vi "LV to ITX 2.2 1D.vi"(0 "Commands":string, 5 "filename":path, 7 "Notes":string, 8 "Array name":string, 9 "1D Array":dbl[](array[numeric])) -> ()   [LabVIEW 2016, in "LV to ITX.lvclass"]
uses:
  LV to ITX.lvclass
panel:
  out "String":string
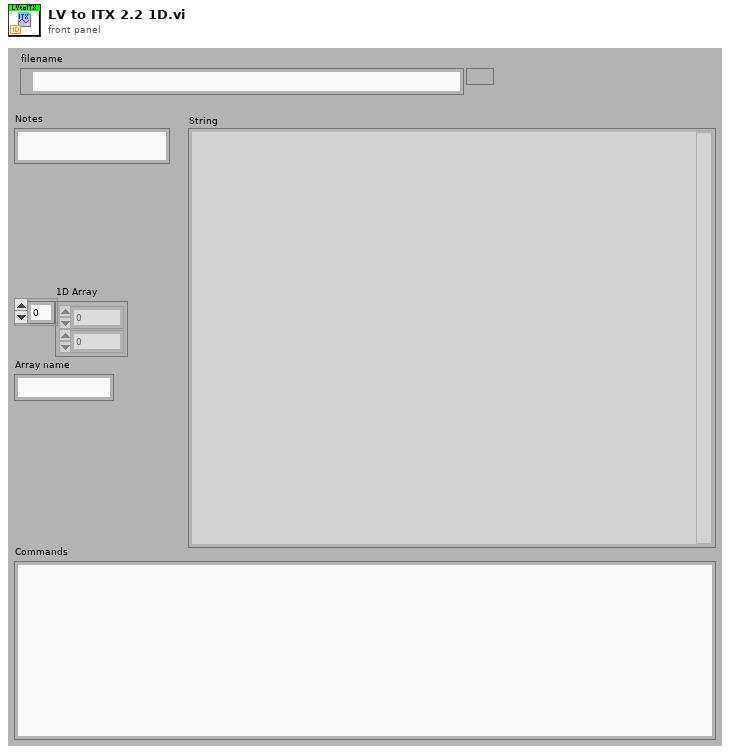
[diagram p1: front panel]
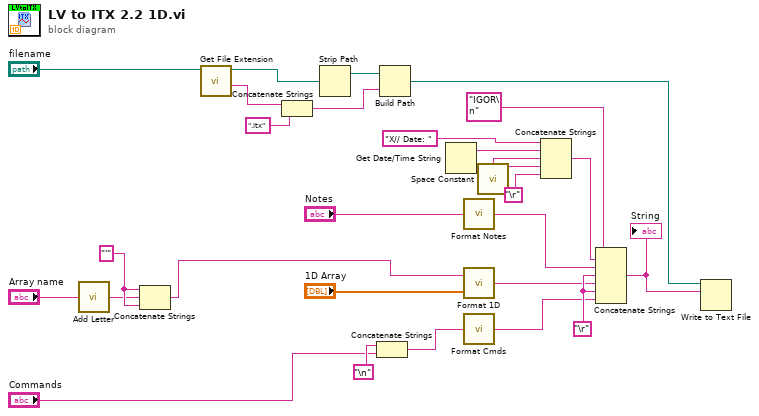
[diagram p0: block diagram]
diagram:
  w3 = "'" ("string")
  w23 = "\r"
  n1 = call "Add Letter.vi"("String"="Array name") -> ("output string"=w2:string)
  n2 = Concatenate Strings(w3, w2, w3) -> (w1:string)
  n3 = call <vilib>:"Get File Extension.vi"("file"="filename") -> ("filename without extension"=w19:string, "dup file"=w15:path)  [unwired: 6 in, 3 out]
  n4 = Concatenate Strings(w19, ".itx") -> (w13:string)
  n5 = Strip Path(path=w15) -> (stripped path=w14:path)  [unwired: 1 out]
  n6 = Concatenate Strings("\n", "Commands") -> (w8:string)
  n7 = Build Path(base path=w14, name or relative path=w13) -> (appended path=w16:path)
  n8 = Get Date/Time String() -> (date string=w27:string, time string=w28:string)  [unwired: 3 in]
  n9 = call "Format Notes.vi"("Notes"="Notes") -> ("String"=w9:string)
  n10 = call "Format 1D.vi"("X 1D Array"="1D Array", "X  Array name"=w1) -> ("String"=w5:string)
  n11 = call "Format Cmds.vi"("Commands"=w8) -> ("String"=w7:string)
  n12 = call <vilib>:"Space Constant.vi"() -> ("String"=w21:string)
  n13 = Concatenate Strings("X// Date: " ("format string"), w27, w21, w28, "\r") -> (w26:string)
  n14 = Concatenate Strings("IGOR\n", w26, w9, w23, w5, w23, w7) -> (w22:string)
  "String" <- w22
  n15 = Write to Text File(file (use dialog)=w16, text=w22) -> ()  [unwired: 2 in, 3 out]
